vi "instrument_error_query.vi"(5 "Beginning error message string (\"\")":string, 7 "Add instrument error to error cluster (T)":bool=TRUE, 8 "error in":errorcluster caption="error in (no error)", 10 "Query (SYST:ERR?)":string="SYST:ERR?", 11 "VISA resource name":refnum<visa-resource-name>) -> (0 "error out":errorcluster, 1 "Error Message(s) out":string, 2 "Error Code":i32, 3 "VISA resource name out":refnum<visa-resource-name>)   [LabVIEW 2022 SP3, in "hmp4000_rsidr_core.lvlib"]
uses:
  hmp4000_rsidr_core.lvlib
  type_Error_Codes.ctl
  Trim Whitespace One-Sided.vi
  Match Regular Expression.xnode
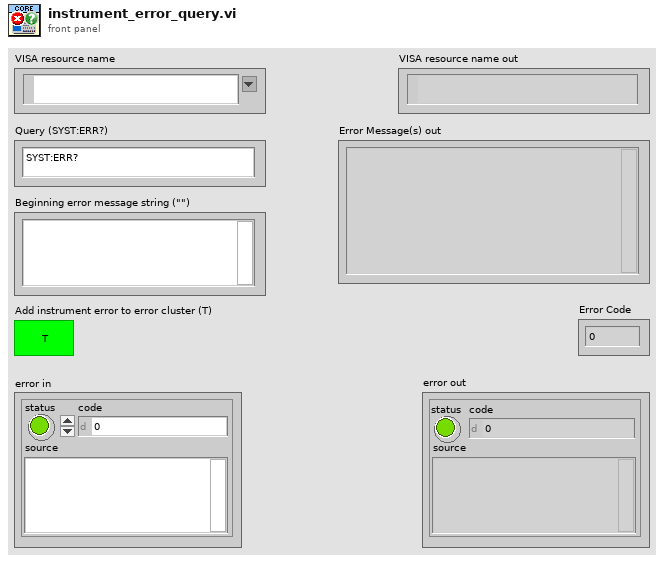
[diagram p1: front panel]
types:
  T1 = typedef "hmp4000_rsidr_core.lvlib/type_Error_Codes.ctl" = enum16{"No_error", "VISA_err_ResourceNotFound", "VISA_err_Timeout", "VISA_warn_MoreDataAvailable", "RS_err_MissingCallback", "RS_err_InvalidAttribute", "RS_err_InvalidValue", "RS_err_UnknownResource", "RS_err_AlreadyInitialized", "RS_err_InstrumentStatus", "RS_err_BadRepCapName", "RS_err_TypesMismatch", "RS_err_ValueNotSupported", "RS_err_InvalidRngTable", "RS_err_IDqueryFail", "RS_err_UnexpResponse", "VISA_warn_ConfigNotLoaded", "RS_err_AttributeNotReadable", "RS_err_AttributeNotWritable", "RS_err_InstrumentType", "RS_err_InstrumentOption", "VISA_err_InvalidSize", "RS_err_ReliabilityIndicator", "VISA_warn_UnknownStatus", "VISA_warn_TermCharRead", "VISA_err_IO_error", "RS_err_FunctionNotSupported", "VISA_warn_QueueEmpty"}
  T2 = typedef "hmp4000_rsidr_core.lvlib/type_Session_Data.ctl" = cluster{"IDN string":string, "Instrument FW":string, "Instr type":string, "Instr type for err. msg.":string, "Installed Options":string[], "Ignore Error Messages":string, "Logging params":variant, "OPC Timeout":i32, "VISA Timeout":i32, "STB Poll VISA Timeout":i32, "Additional Flags":i32, "Wait Before Read":i32, "Wait Before Write":i32, "Option String Flags":i32, "IO Segment Size":i64, "VISA Access Mode":T3, "Interface Type":T4, "OPC Wait Mode":T5, "Bin Float Number  Format":T6, "Bin Integer Number Format":T7, "Simulate":bool, "VXIcapable":bool, "Duplicate Session":bool, "Add LF to Write":bool, "Logging":bool, "Fast Sweep":bool, "Query Instrument Status":bool, "Check Range":bool, "Check Options":bool}
  T3 = typedef "hmp4000_rsidr_core.lvlib/type_VisaAccessMode.ctl" = u16
  T4 = typedef "hmp4000_rsidr_core.lvlib/type_InterfaceType.ctl" = enum16{"Unknown", "GPIB", "VXI", "GPIB_VXI", "ASRL", "PXI", "TCPIP", "USB", "SOCKET"}
  T5 = typedef "hmp4000_rsidr_core.lvlib/type_OPC_Wait_Mode.ctl" = enum16{"STBpolling", "STBpollingSlow", "STBpollingSuperSlow", "ServiceRequest", "OPCquery"}
  T6 = typedef "hmp4000_rsidr_core.lvlib/type_Binary_Float_Number_Format.ctl" = enum16{"Float_4_Bytes_Swapped", "Float_4_Bytes", "Double_8_Bytes_Swapped", "Double_8_Bytes"}
  T7 = typedef "hmp4000_rsidr_core.lvlib/type_Binary_Integer_Number_Format.ctl" = enum16{"Int32_4_Bytes_Swapped", "Int32_4 Bytes", "Int16_2_Bytes_Swapped", "Int16_2_Bytes"}
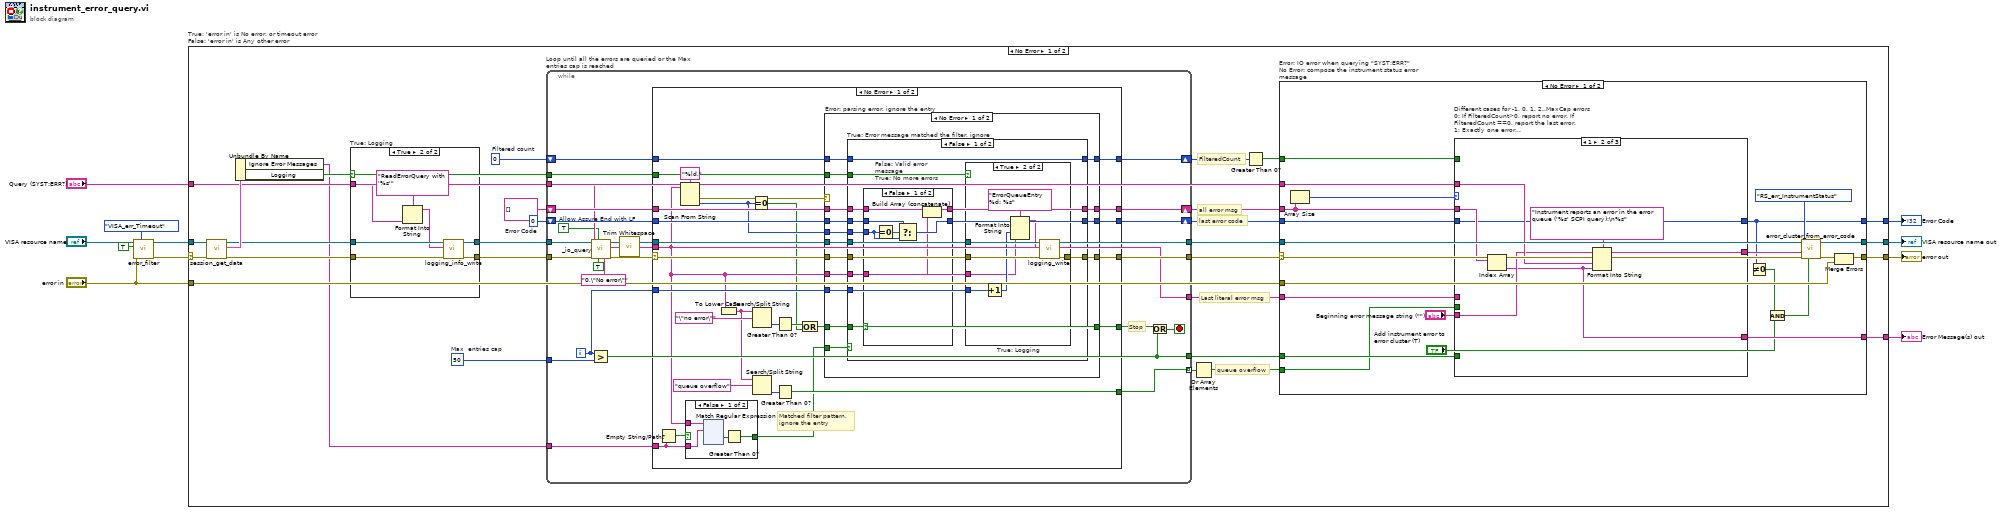
[diagram p0: block diagram]
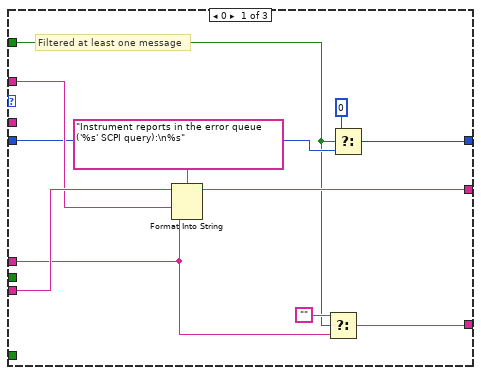
[diagram p3: hidden frame]
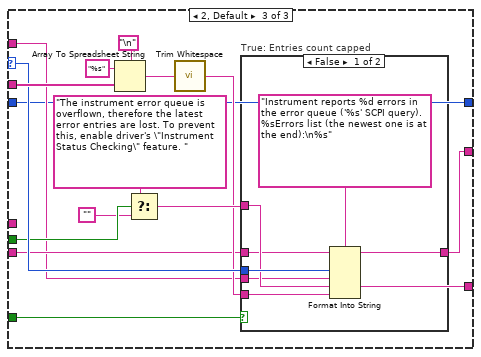
[diagram p4: hidden frame]
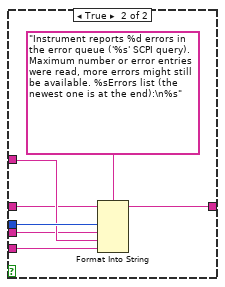
[diagram p5: hidden frame]
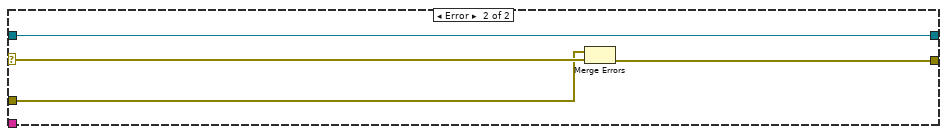
[diagram p6: hidden frame]
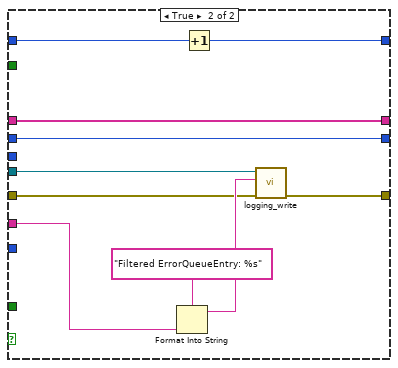
[diagram p9: hidden frame]
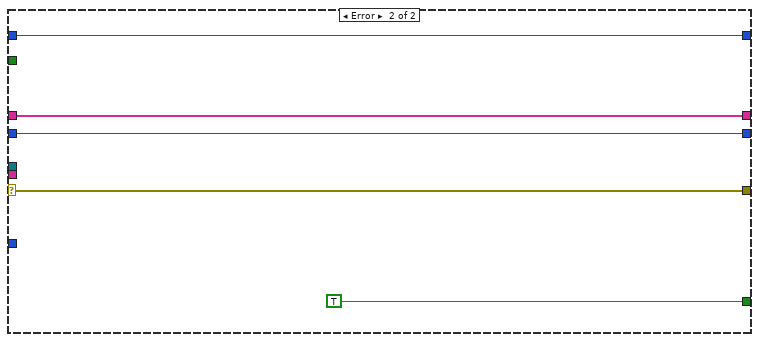
[diagram p12: hidden frame]
diagram:
  n1 = call "error_filter.vi"("Error Enum in"=type_Error_Codes."VISA_err_Timeout" ("Code to detect"), "error in"="error in", "Clear detected code (F)"=TRUE ("Clear detected error (F)"), "VISA resource name"="VISA resource name") -> ("error out"=w5:errorcluster, "VISA resource name out"=w2:refnum<visa-resource-name>)  [unwired: 5 in, 1 out]
  n2 = case "True: 'error in' is No error, or timeout error\nFalse: 'error in' is Any other error" shown="No Error" w5 {
    selector: w5 -> [w24 _]
    tunnel: [w33 _] -> w9
    tunnel: [w35 _] -> w11
    tunnel: [w19 w363] -> w8
    tunnel: w2 -> [w25 w363]
    tunnel: "error in" -> [w28 w362]
    tunnel: [w27 w362] -> w10
    tunnel: "Query (SYST:ERR?)" -> [w16 _]
    frame No Error {
      w14 = 0  # Filtered count
      w32 = 50  # Max  entries cap
      w39 = 0  # Error Code
      # "FilteredCount"
      # "queue overflow"
      # "Last literal error msg"
      # "last error code"
      # "all error msg"
      n3 = call "session_get_data.vi"("error in"=w24, "VISA resource name"=w25) -> ("error out"=w21:errorcluster, "Session User Data out"=w23:T2, "VISA resource name out"=w22:refnum<visa-resource-name>)  [unwired: 6 in, 1 out]
      n4 = Unbundle By Name(w23) -> ("Ignore Error Messages"=w15:string, "Logging"=w20:bool)
      n5 = case "True: Logging" shown="True" w20 {
        tunnel: w22 -> [w42 w49]
        tunnel: [w42 w48] -> w18
        tunnel: w21 -> [w41 w47]
        tunnel: [w41 w46] -> w17
        tunnel: w16 -> [_ w44]
        frame False {
        }
        frame True {
          n6 = Format Into String(format string="ReadErrorQuery with '%s'" ("String to write"), w44) -> (resulting string=w43:string)  [unwired: 2 in, 1 out]
          n7 = call "logging_info_write.vi"("error in"=w47, "String to write"=w43, "VISA resource name"=w49) -> ("error out"=w46:errorcluster, "VISA resource name out"=w48:refnum<visa-resource-name>)  [unwired: 7 in]
        }
      }
      n8 = while "Loop until all the errors are queried or the Max  entries cap is reached" {
        tunnel: [w135] -> w26
        tunnel: w18 -> [w136]
        tunnel: [w134] -> w36
        shift-right: [w146] -> w38
        shift-left: string[] [] -> [w147]
        shift-right: [w144] -> w37
        shift-left: w39 -> [w145]
        tunnel: [w124] -> w34
        tunnel: w32 -> [w141]
        tunnel: [w140] -> w31
        tunnel: [w139] -> w30 mode=indexing
        tunnel: w17 -> [w137]
        tunnel: w20 -> [w133]
        tunnel: w16 -> [w129]
        tunnel: w15 -> [w128]
        shift-right: [w126] -> w13
        shift-left: w14 -> [w127]
        i -> [w132]
        stop <- w142 stop-if-true
        w123 = TRUE  # Allow Assure End with LF
        # "Stop"
        n9 = call "_io_query.vi"("Simulation read buffer (\"Simulation\")"="0,\"No error\"" ("Simulation read buffer \n(\"Simulation\")"), "Block Logging (F)"=TRUE, "Allow Assure End with LF"=w123, "error in"=w137, "Write buffer"=w129, "VISA resource name"=w136) -> ("error out"=w138:errorcluster, "Read buffer"=w125:string, "VISA resource name out"=w135:refnum<visa-resource-name>)  [unwired: 2 in, 1 out]
        n10 = Greater?(x=w132, y=w141) -> (0:w140:bool)
        n11 = call "Trim Whitespace.vi"("string"=w125) -> ("trimmed string"=w124:string)  [unwired: 1 in]
        n12 = case shown="No Error" w138 {
          selector: w138 -> [w163 w358]
          tunnel: [w148 TRUE] -> w143
          tunnel: w147 -> [w171 w361]
          tunnel: [w170 w361] -> w146
          tunnel: w145 -> [w169 w360]
          tunnel: [w168 w360] -> w144
          tunnel: [w164 _] -> w139
          tunnel: w135 -> [w162 _]
          tunnel: [w161 w358] -> w134
          tunnel: w133 -> [w160 _]
          tunnel: w132 -> [w159 _]
          tunnel: w128 -> [w153 _]
          tunnel: w127 -> [w155 w357]
          tunnel: [w154 w357] -> w126
          tunnel: w124 -> [w152 _]
          frame No Error {
            # "Matched filter pattern,\nignore the entry"
            n13 = Empty String/Path?(string/path=w153) -> (empty?=w157:bool)
            n14 = Scan From String(format string="%ld,", input string=w152) -> (error out=w149:errorcluster, output 1=w151:i32)  [unwired: 3 in, 2 out]
            n15 = case shown="False" w157 {
              tunnel: w153 -> [w238 _]
              tunnel: w152 -> [w239 _]
              tunnel: [w236 _] -> w156
              frame False {
                n16 = xnode "Match Regular Expression"("input string"=w239, "regular expression"=w238) -> ("offset past match"=w237:i32)  [unwired: 4 in, 4 out]
                n17 = Greater Than 0?(x=w237) -> (x > 0?=w236:bool)
              }
              frame True {
              }
            }
            n18 = To Lower Case(string=w152) -> (all lower case string=w167:string)
            n19 = Equal To 0?(x=w151) -> (x = 0?=w150:bool)
            n20 = Search/Split String(string=w167, search string/char (-)="\"no error\"") -> (offset of match=w173:i32)  [unwired: 1 in, 2 out]
            n21 = Search/Split String(string=w167, search string/char (-)="queue overflow") -> (offset of match=w165:i32)  [unwired: 1 in, 2 out]
            n22 = Greater Than 0?(x=w173) -> (x > 0?=w158:bool)
            n23 = Greater Than 0?(x=w165) -> (x > 0?=w164:bool)
            n24 = Compound Arithmetic op=OR(w158, w150) -> (w172:bool)
            n25 = case "Error: parsing error, ignore the entry" shown="No Error" w149 {
              tunnel: w172 -> [w176 _]
              tunnel: w171 -> [w190 w235]
              tunnel: [w189 w235] -> w170
              tunnel: w169 -> [w188 w234]
              tunnel: [w187 w234] -> w168
              tunnel: w163 -> [w186 w233]
              tunnel: w162 -> [w185 _]
              tunnel: [w184 w233] -> w161
              tunnel: w160 -> [w183 _]
              tunnel: w159 -> [w182 _]
              tunnel: w156 -> [w181 _]
              tunnel: w155 -> [w180 w232]
              tunnel: [w179 w232] -> w154
              tunnel: w152 -> [w178 _]
              tunnel: w151 -> [w177 _]
              tunnel: [w176 _] -> w148
              frame No Error {
                n26 = case "True: Error message matched the filter, ignore" shown="False" w181 {
                  tunnel: w176 -> [w203 _]
                  tunnel: w190 -> [w202 w231]
                  tunnel: [w201 w231] -> w189
                  tunnel: w177 -> [w200 _]
                  tunnel: w188 -> [w199 w230]
                  tunnel: [w198 w230] -> w187
                  tunnel: w186 -> [w197 w225]
                  tunnel: w185 -> [w196 w224]
                  tunnel: [w195 w222] -> w184
                  tunnel: w183 -> [w194 _]
                  tunnel: w182 -> [w193 _]
                  tunnel: w178 -> [w191 w223]
                  tunnel: w180 -> [w192 w229]
                  tunnel: [w192 w228] -> w179
                  frame False {
                    n27 = case "False: Valid error message\nTrue: No more errors" shown="False" w203 {
                      tunnel: w202 -> [w218 w221]
                      tunnel: [w219 w221] -> w201
                      tunnel: w200 -> [w214 _]
                      tunnel: w199 -> [w216 w220]
                      tunnel: [w215 w220] -> w198
                      tunnel: w191 -> [w213 _]
                      frame False {
                        n28 = Equal To 0?(x=w214) -> (x = 0?=w217:bool)
                        n29 = Select(t=w216, s=w217, f=w214) -> (s? t:f=w215:i32)
                        n30 = Build Array (concatenate)(w218, w213) -> (w219:string[])
                      }
                      frame True {
                      }
                    }
                    n31 = case "True: Logging" shown="True" w194 {
                      tunnel: w197 -> [w204 w212]
                      tunnel: w196 -> [_ w211]
                      tunnel: [w204 w210] -> w195
                      tunnel: w193 -> [_ w207]
                      tunnel: w191 -> [_ w205]
                      frame False {
                      }
                      frame True {
                        n32 = Increment(x=w207) -> (x+1=w206:i32)
                        n33 = Format Into String(format string="ErrorQueueEntry %d: %s", w206, w205) -> (resulting string=w209:string)  [unwired: 2 in, 1 out]
                        n34 = call "logging_write.vi"("error in"=w212, "String to write"=w209, "VISA resource name"=w211) -> ("error out"=w210:errorcluster)  [unwired: 7 in, 1 out]
                      }
                    }
                  }
                  frame True {
                    n35 = Format Into String(format string="Filtered ErrorQueueEntry: %s", w223) -> (resulting string=w227:string)  [unwired: 2 in, 1 out]
                    n36 = Increment(x=w229) -> (x+1=w228:i32)
                    n37 = call "logging_write.vi"("error in"=w225, "String to write"=w227, "VISA resource name"=w224) -> ("error out"=w222:errorcluster)  [unwired: 7 in, 1 out]
                  }
                }
              }
              frame Error {
              }
            }
          }
          frame Error {
          }
        }
        n38 = Or(x=w143, y=w140) -> (x .or. y?=w142:bool)
      }
      n39 = Or Array Elements(Boolean array=w30) -> (logical OR=w29:bool)
      n40 = Greater Than 0?(x=w13) -> (x > 0?=w12:bool)
      n41 = case "Error: IO error when querying \"SYST:ERR?\"\nNo Error: compose the instrument status error message" shown="No Error" w36 {
        selector: w36 -> [w60 w122]
        tunnel: [w65 w120] -> w27
        tunnel: [w69 _] -> w33
        tunnel: [w52 _] -> w35
        tunnel: w38 -> [w71 _]
        tunnel: w37 -> [w53 _]
        tunnel: w34 -> [w70 _]
        tunnel: w31 -> [w68 _]
        tunnel: w29 -> [w67 _]
        tunnel: w28 -> [w64 w121]
        tunnel: w26 -> [w59 w119]
        tunnel: [w63 w119] -> w19
        tunnel: w16 -> [w54 _]
        tunnel: w12 -> [w50 _]
        frame No Error {
          n42 = Array Size(array=w71) -> (size(s)=w51:i32)
          n43 = case "Different cases for -1, 0, 1, 2..MaxCap errors\n0: If FilteredCount>0, report no error. If FilteredCount ==0, report the last error.\n1: Exactly one error\n2, Default: 2 or more messages" shown="1" w51 {
            selector: w51 -> [_ _ w102]
            tunnel: [w79 w88 w103] -> w61
            tunnel: w71 -> [_ w84 w104]
            tunnel: w70 -> [w77 _ _]
            tunnel: [w78 w85 w93] -> w69
            tunnel: w68 -> [_ _ w98]
            tunnel: w67 -> [_ _ w97]
            tunnel: "Beginning error message string (\"\")" -> [w81 w86 w92]
            tunnel: w54 -> [w80 w87 w91]
            tunnel: w53 -> [w75 w83 w90]
            tunnel: [w73 w83 w90] -> w52
            tunnel: w50 -> [w74 _ _]
            frame 0 {
              # "Filtered at least one message"
              n44 = Format Into String(format string="Instrument reports in the error queue ('%s' SCPI query):\n%s" ("Source"), initial string=w81, w80, w77) -> (resulting string=w79:string)  [unwired: 1 in, 1 out]
              n45 = Select(t="", s=w74, f=w77) -> (s? t:f=w78:string)
              n46 = Select(t=0, s=w74, f=w75) -> (s? t:f=w73:i32)
            }
            frame 1 {
              n47 = Index Array(array=w84) -> (element=w85:string)  [unwired: 1 in]
              n48 = Format Into String(format string="Instrument reports an error in the error queue ('%s' SCPI query):\n%s" ("Source"), initial string=w86, w87, w85) -> (resulting string=w88:string)  [unwired: 1 in, 1 out]
            }
            frame 2, Default {
              n49 = Array To Spreadsheet String(delimiter (Tab)="\n" ("Line Feed Constant"), array=w104, 3:"%s" ("format string")) -> (spreadsheet string=w99:string)
              n50 = Select(t="The instrument error queue is overflown, therefore the latest error entries are lost. To prevent this, enable driver's \"Instrument Status Checking\" feature. " ("Source"), s=w97, f="" ("Empty String Constant")) -> (s? t:f=w94:string)
              n51 = call "Trim Whitespace.vi"("string"=w99) -> ("trimmed string"=w93:string)  [unwired: 1 in]
              n52 = case "True: Entries count capped" shown="False" w98 {
                tunnel: [w110 w117] -> w103
                tunnel: w102 -> [w109 w116]
                tunnel: w93 -> [w108 w115]
                tunnel: w94 -> [w107 w114]
                tunnel: w92 -> [w106 w113]
                tunnel: w91 -> [w105 w112]
                frame False {
                  n53 = Format Into String(format string="Instrument reports %d errors in the error queue ('%s' SCPI query). %sErrors list (the newest one is at the end):\n%s" ("Source"), initial string=w106, w109, w105, w107, w108) -> (resulting string=w110:string)  [unwired: 1 in, 1 out]
                }
                frame True {
                  n54 = Format Into String(format string="Instrument reports %d errors in the error queue ('%s' SCPI query). Maximum number or error entries were read, more errors might still be available. %sErrors list (the newest one is at the end):\n%s" ("Source"), initial string=w113, w116, w112, w114, w115) -> (resulting string=w117:string)  [unwired: 1 in, 1 out]
                }
              }
            }
          }
          n55 = Not Equal To 0?(x=w52) -> (x != 0?=w58:bool)
          n56 = Compound Arithmetic op=AND(w58, "Add instrument error to error cluster (T)") -> (w56:bool)
          n57 = call "error_cluster_from_error_code.vi"("Error Creation Enabled (True)"=w56, "error in"=w60, "Error Message (\"\")"=w61, "Error Enum in"=type_Error_Codes."RS_err_InstrumentStatus", "VISA resource name"=w59) -> ("error out"=w66:errorcluster, "VISA resource name out"=w63:refnum<visa-resource-name>)  [unwired: 5 in]
          n58 = Merge Errors(w66, w64) -> (w65:errorcluster)
        }
        frame Error {
          n59 = Merge Errors(w121, w122) -> (w120:errorcluster)
        }
      }
    }
    frame Error {
    }
  }
  "Error Message(s) out" <- w9
  "Error Code" <- w11
  "VISA resource name out" <- w8
  "error out" <- w10
